vi "DAC_set_slot-timings.vi"(8 "Time (ms)":T1 min=-1 max=0.5, 10 "slot number":u16, 11 "FPGA VI Reference In":T2) -> (3 "FPGA VI Reference Out":T2)   [LabVIEW 2013]
uses:
  fpga-bitfile-ref.ctl
  sequence slot/DAC_fastseq-offset.ctl
  slot-use-type.ctl
  slot-use-values.ctl
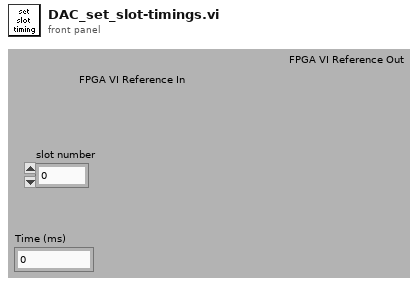
[diagram p1: front panel]
types:
  T1 = typedef "DAC_fastseq-offset.ctl" = sgl
  T2 = typedef "fpga-bitfile-ref.ctl" = refnum<k20>
  T3 = typedef "slot-use-values.ctl" = enum16{"DAC", "timing", "triggers", "jump"}
  T4 = typedef "slot-use-type.ctl" = fxp<+,4,4>
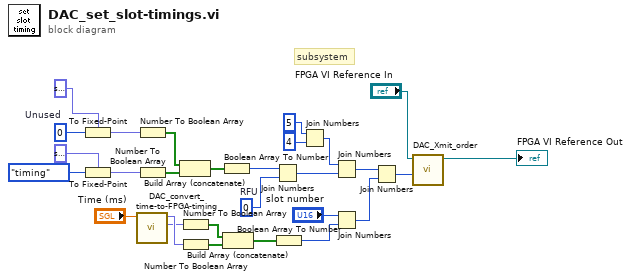
[diagram p0: block diagram]
diagram:
  w12 = u8 0  # Unused
  w25 = u8 0  # RFU
  # "subsystem"
  n1 = To Fixed-Point(fixed-point type=T4 0.0, number=w12) -> (fixed-point=w17:T4)
  n2 = To Fixed-Point(fixed-point type=T4 0.0, number=slot-use-values."timing") -> (fixed-point=w16:T4)
  n3 = call "DAC_convert_time-to-FPGA-timing.vi"("time (ms)"="Time (ms)") -> ("p"=w3:fxp<+,11,11>, "n"=w4:fxp<+,5,5>)  [unwired: 9 out]
  n4 = Number To Boolean Array(number=w17) -> (Boolean array=w1:bool[])
  n5 = Number To Boolean Array(number=w16) -> (Boolean array=w2:bool[])
  n6 = Build Array (concatenate)(w1, w2) -> (w18:bool[])
  n7 = Number To Boolean Array(number=w3) -> (Boolean array=w9:bool[])
  n8 = Number To Boolean Array(number=w4) -> (Boolean array=w8:bool[])
  n9 = Boolean Array To Number(Boolean array=w18) -> (number=w10:u8)
  n10 = Build Array (concatenate)(w9, w8) -> (w7:bool[])
  n11 = Join Numbers(hi=w10, lo=w25) -> ((hi.lo)=w24:u16)
  n12 = Boolean Array To Number(Boolean array=w7) -> (number=w6:u16)
  n13 = Join Numbers(hi=u8 5, lo=u8 4) -> ((hi.lo)=w23:u16)
  n14 = Join Numbers(hi=w23, lo=w24) -> ((hi.lo)=w20:u32)
  n15 = Join Numbers(hi="slot number", lo=w6) -> ((hi.lo)=w21:u32)
  n16 = Join Numbers(hi=w20, lo=w21) -> ((hi.lo)=w28:u64)
  n17 = call "DAC_Xmit_order.vi"("Order in"=w28, "FPGA VI Reference In"="FPGA VI Reference In") -> ("FPGA VI Reference Out"=→"FPGA VI Reference Out":T2)  [unwired: 9 out]
